vi "409b_SuperTable2.vi"(1 "Port":refnum<visa-resource-name>="COM1", 2 "Table":string[][](table)=[["1", "0000", "89.75", "0", "100", "ff"], ["0", "0000", "89.75", "0", "100", "ff"], ["1", "0001", "90.25", "0", "100", "00"], ["0", "0001", "90.25", "0", "100", "00"], ["", "", "", "", "", ""], ["", "", "", "", "", ""]] caption="Commands") -> (0 "Results2":string[][](table) caption="Results")   [LabVIEW 2013]
panel:
  in  "Intermediate":string[][](table) caption="intermediate"
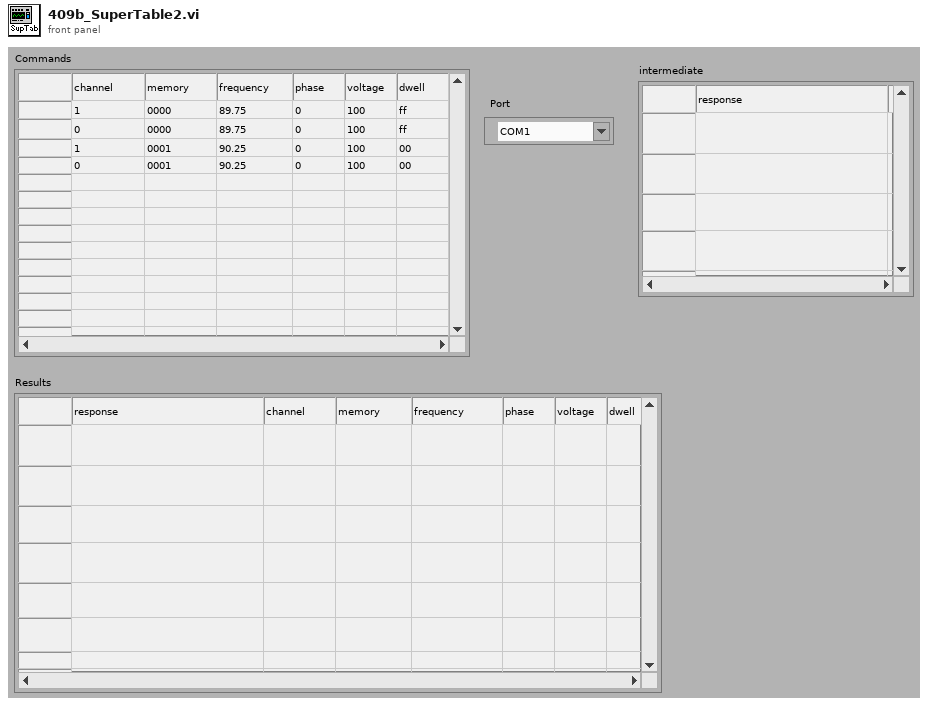
[diagram p1: front panel]
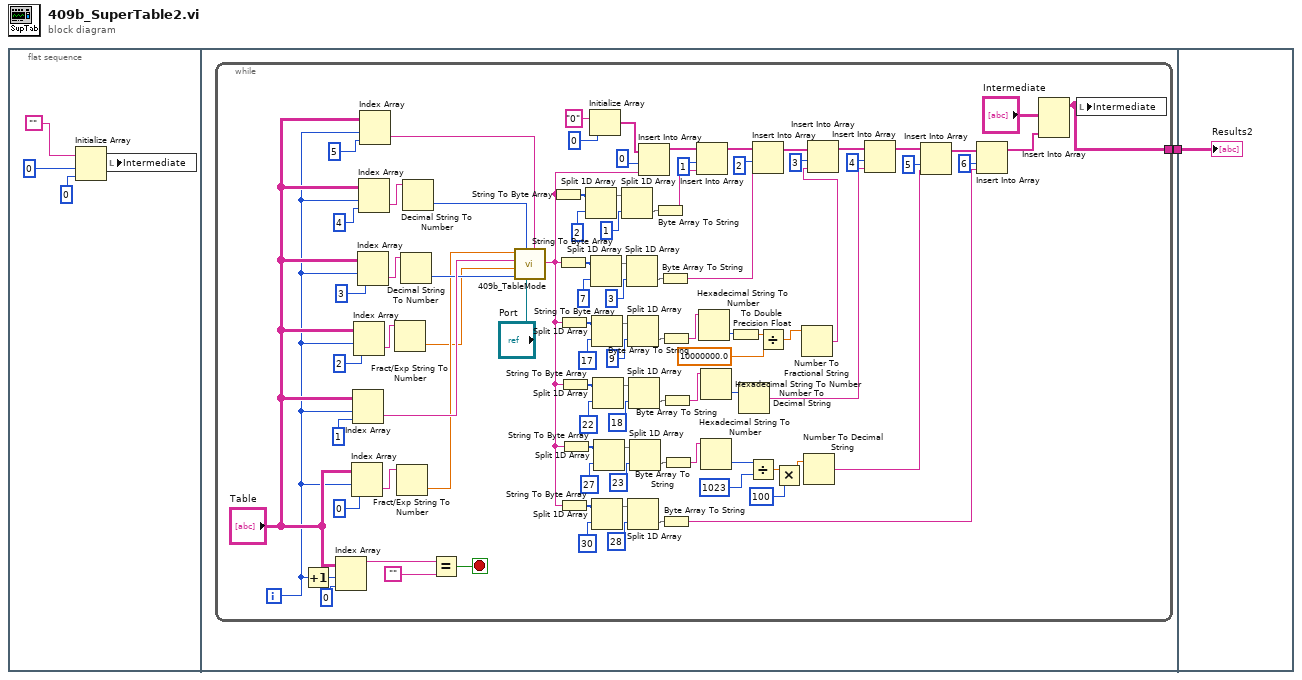
[diagram p0: block diagram]
diagram:
  n1 = flat-sequence {
    tunnel: [w6] -> w1
    tunnel: w1 -> [w100]
    frame #0 {
      n2 = Initialize Array("", 0, 0) -> (w3:string[][])
      n3 = local write "Intermediate"(w3) -> ()
    }
    frame #1 {
      n4 = while {
        tunnel: [w7] -> w6
        i -> [w18]
        stop <- w96 stop-if-true
        n5 = Increment(x=w18) -> (x+1=w82:i32)
        n6 = Index Array(array="Table", index (row)=w82, index (col)=0) -> (element=w98:string)
        n7 = Index Array(array="Table", index (row)=w18, index (col)=0) -> (element=w15:string)
        n8 = Index Array(array="Table", index (row)=w18, index (col)=1) -> (element=w89:string)
        n9 = Index Array(array="Table", index (row)=w18, index (col)=2) -> (element=w13:string)
        n10 = Index Array(array="Table", index (row)=w18, index (col)=3) -> (element=w87:string)
        n11 = Index Array(array="Table", index (row)=w18, index (col)=4) -> (element=w85:string)
        n12 = Index Array(array="Table", index (row)=w18, index (col)=5) -> (element=w88:string)
        n13 = Fract/Exp String To Number(string=w13) -> (number=w12:dbl)  [unwired: 3 in, 1 out]
        n14 = Fract/Exp String To Number(string=w15) -> (number=w14:dbl)  [unwired: 3 in, 1 out]
        n15 = Decimal String To Number(string=w87) -> (number=w86:i32)  [unwired: 2 in, 1 out]
        n16 = Decimal String To Number(string=w85) -> (number=w84:i32)  [unwired: 2 in, 1 out]
        n17 = Equal?(x=w98, y="") -> (x = y?=w96:bool)
        n18 = call "409b_TableMode.vi"("Dwell (Hex)"=w88, "Port"="Port", "Voltage"=w84, "Phase"=w86, "Frequency (MHz)"=w12, "Memory (Hex)"=w89, "Channel"=w14) -> ("Confirm"=w31:string)  [unwired: 2 in, 2 out]
        n19 = String To Byte Array(string=w31) -> (unsigned byte array=w75:u8[])
        n20 = String To Byte Array(string=w31) -> (unsigned byte array=w67:u8[])
        n21 = String To Byte Array(string=w31) -> (unsigned byte array=w59:u8[])
        n22 = String To Byte Array(string=w31) -> (unsigned byte array=w40:u8[])
        n23 = String To Byte Array(string=w31) -> (unsigned byte array=w54:u8[])
        n24 = String To Byte Array(string=w31) -> (unsigned byte array=w45:u8[])
        n25 = Split 1D Array(array=w75, index=2) -> (first subarray=w69:u8[])  [unwired: 1 out]
        n26 = Initialize Array("0", 0) -> (w76:string[])
        n27 = Split 1D Array(array=w67, index=7) -> (first subarray=w64:u8[])  [unwired: 1 out]
        n28 = Split 1D Array(array=w59, index=17) -> (first subarray=w56:u8[])  [unwired: 1 out]
        n29 = Split 1D Array(array=w40, index=30) -> (first subarray=w37:u8[])  [unwired: 1 out]
        n30 = Split 1D Array(array=w54, index=22) -> (first subarray=w51:u8[])  [unwired: 1 out]
        n31 = Split 1D Array(array=w45, index=27) -> (first subarray=w42:u8[])  [unwired: 1 out]
        n32 = Split 1D Array(array=w69, index=1) -> (second subarray=w68:u8[])  [unwired: 1 out]
        n33 = Split 1D Array(array=w64, index=3) -> (second subarray=w63:u8[])  [unwired: 1 out]
        n34 = Split 1D Array(array=w56, index=9) -> (second subarray=w55:u8[])  [unwired: 1 out]
        n35 = Split 1D Array(array=w37, index=28) -> (second subarray=w36:u8[])  [unwired: 1 out]
        n36 = Split 1D Array(array=w51, index=18) -> (second subarray=w50:u8[])  [unwired: 1 out]
        n37 = Split 1D Array(array=w42, index=23) -> (second subarray=w41:u8[])  [unwired: 1 out]
        n38 = Insert Into Array(array=w76, index=0, new element=w31) -> (w71:string[])
        n39 = Byte Array To String(unsigned byte array=w68) -> (string=w72:string)
        n40 = Byte Array To String(unsigned byte array=w63) -> (string=w60:string)
        n41 = Byte Array To String(unsigned byte array=w55) -> (string=w9:string)
        n42 = Byte Array To String(unsigned byte array=w36) -> (string=w30:string)
        n43 = Byte Array To String(unsigned byte array=w50) -> (string=w28:string)
        n44 = Byte Array To String(unsigned byte array=w41) -> (string=w25:string)
        n45 = Insert Into Array(array=w71, index=1, new element=w72) -> (w61:string[])
        n46 = Hexadecimal String To Number(string=w9) -> (number=w8:u32)  [unwired: 2 in, 1 out]
        n47 = Hexadecimal String To Number(string=w28) -> (number=w27:u32)  [unwired: 2 in, 1 out]
        n48 = Hexadecimal String To Number(string=w25) -> (number=w23:u32)  [unwired: 2 in, 1 out]
        n49 = To Double Precision Float(number=w8) -> (double precision float=w17:dbl)
        n50 = Number To Decimal String(number=w27) -> (decimal integer string=w26:string)  [unwired: 1 in]
        n51 = Divide(x=w23, y=1023) -> (x/y=w19:dbl)
        n52 = Insert Into Array(array=w61, index=2, new element=w60) -> (w48:string[])
        n53 = Divide(x=w17, y=10000000.0) -> (x/y=w11:dbl)
        n54 = Multiply(x=w19, y=100) -> (x*y=w21:dbl)
        n55 = Number To Fractional String(number=w11) -> (F-format string=w10:string)  [unwired: 3 in]
        n56 = Number To Decimal String(number=w21) -> (decimal integer string=w24:string)  [unwired: 1 in]
        n57 = Insert Into Array(array=w48, index=3, new element=w10) -> (w46:string[])
        n58 = Insert Into Array(array=w46, index=4, new element=w26) -> (w33:string[])
        n59 = Insert Into Array(array=w33, index=5, new element=w24) -> (w32:string[])
        n60 = Insert Into Array(array=w32, index=6, new element=w30) -> (w29:string[])
        n61 = Insert Into Array(array="Intermediate", new element=w29) -> (w7:string[][])  [unwired: 2 in]
        n62 = local write "Intermediate"(w7) -> ()
      }
    }
    frame #2 {
      "Results2" <- w100
    }
  }
